vi "PC.vi"() -> ()   [LabVIEW 2016]
uses:
  <vilib>/addons/database/Connection.llb/DB Tools Open Connec (Path).vi
  <vilib>/addons/database/NI_Database_API.lvlib
panel:
  in  "stop 2":bool
  in  "connection information":path
  out "Array 2":dbl[][](array[numeric])
  in  "stop":bool
  in  "kl2":bool
  in  "Reset timer 2":bool
  out "Timer2":u32
  in  "kl1":bool
  in  "Reset timer 1":bool
  out "Timer1":u32
  in  "kl0":bool
  out "Timer0":u32
  in  "Reset timer":bool
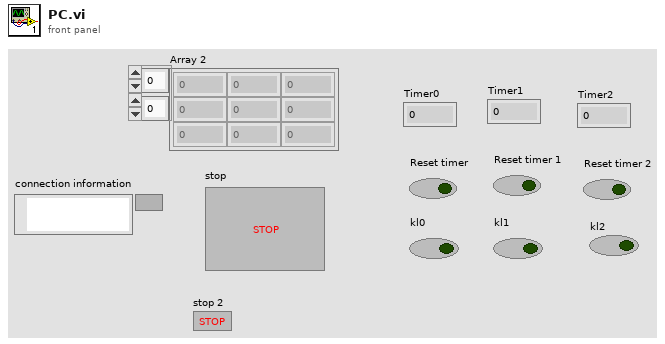
[diagram p1: front panel]
types:
  T1 = cluster{"Place1":string, "Place2":string, "Place3":string}
  T2 = typedef "NI_Database_API.lvlib/Conn ObjectReference.ctl" = refnum<k1>
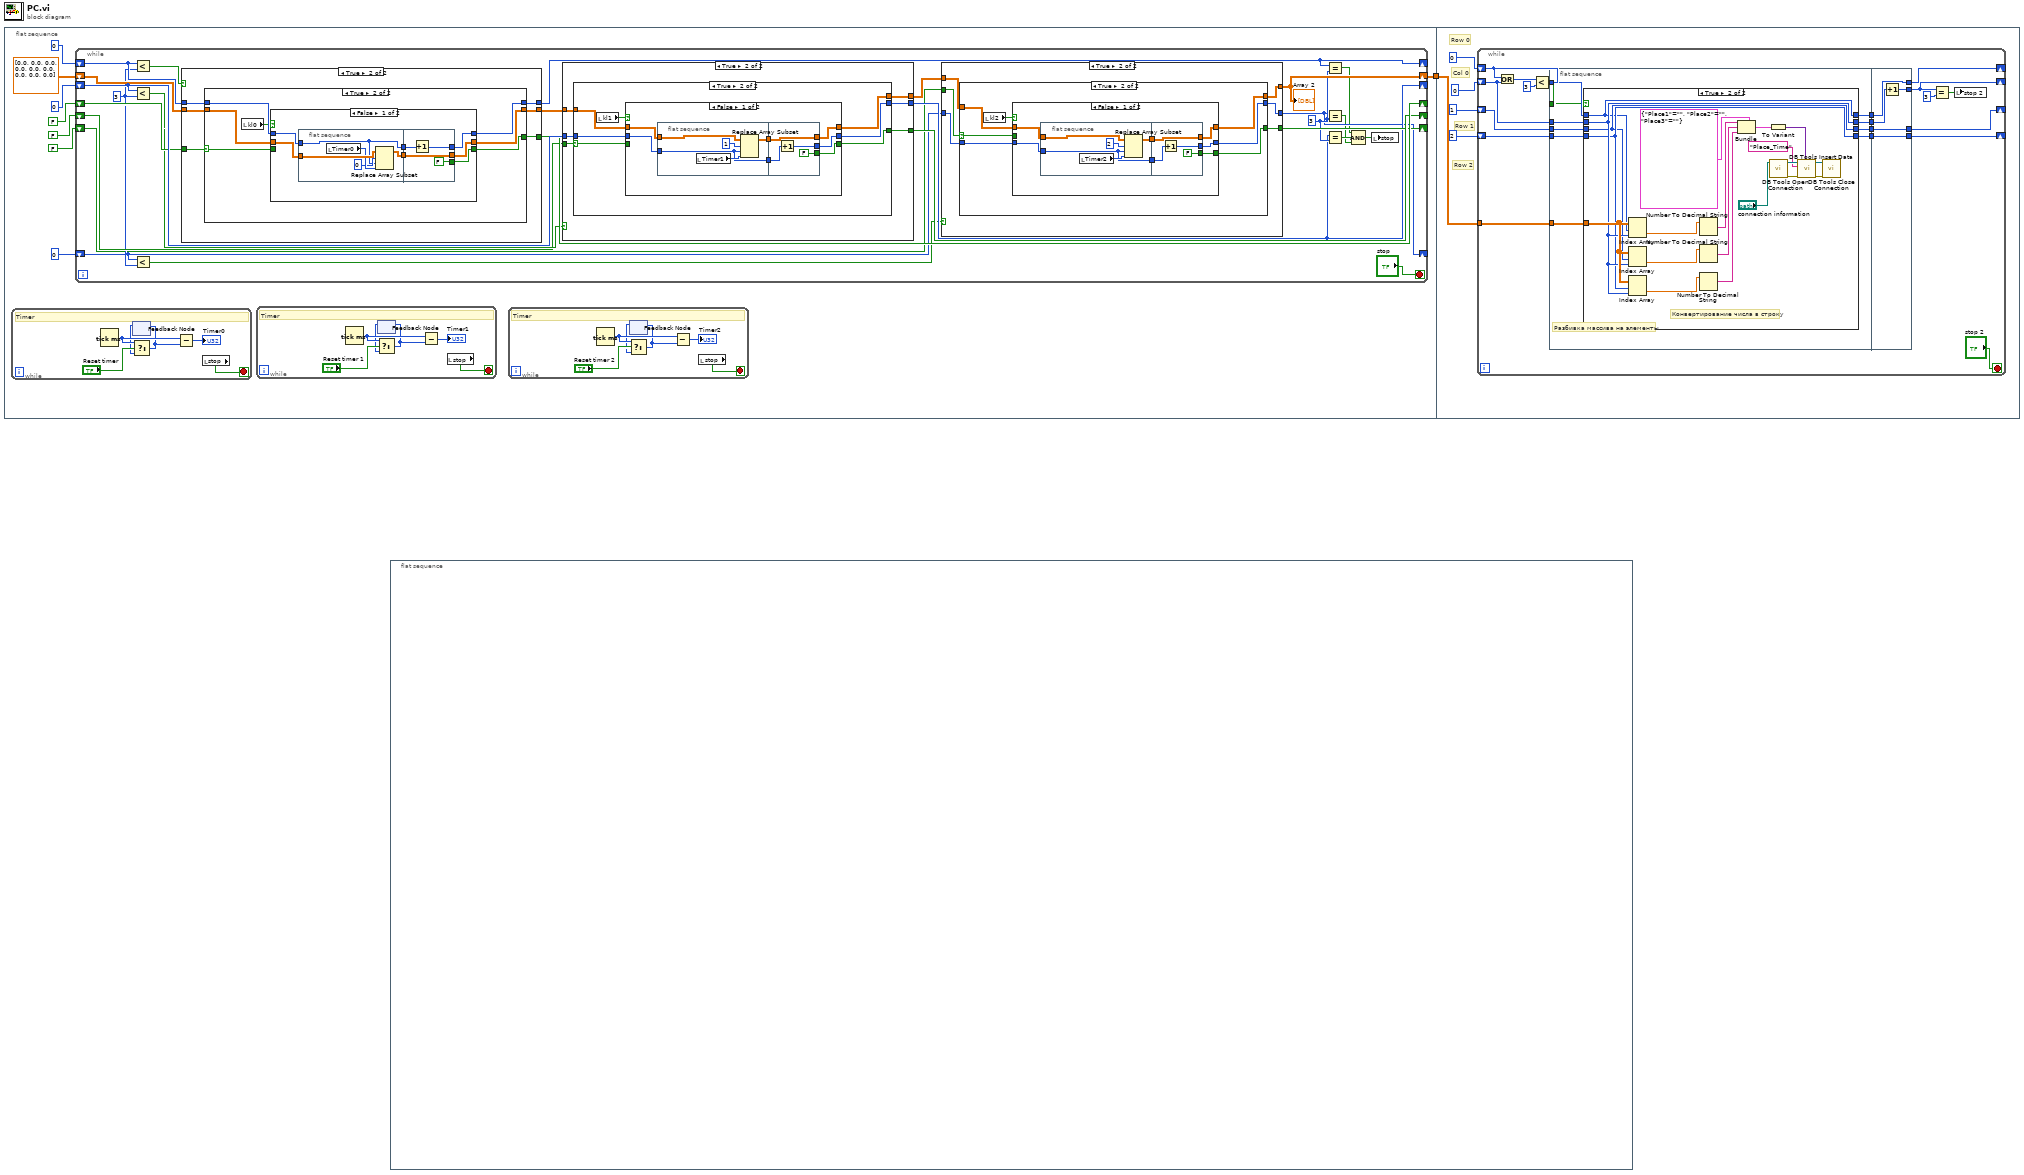
[diagram p0: block diagram]
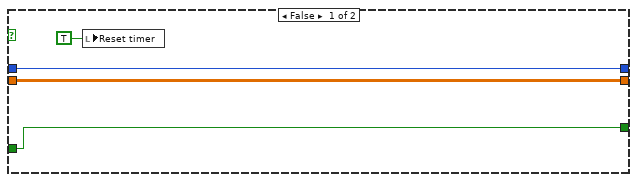
[diagram p2: hidden frame]
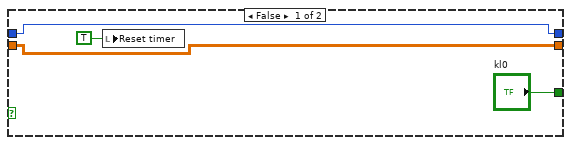
[diagram p3: hidden frame]
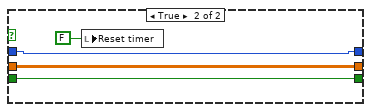
[diagram p4: hidden frame]
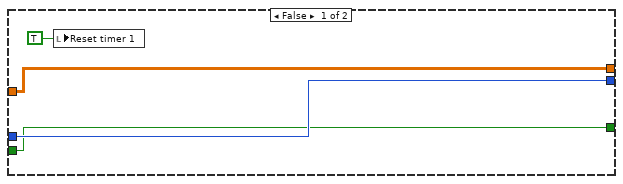
[diagram p5: hidden frame]
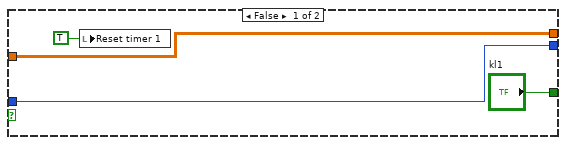
[diagram p6: hidden frame]
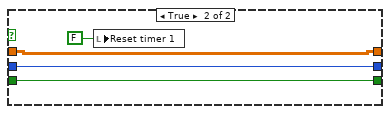
[diagram p7: hidden frame]
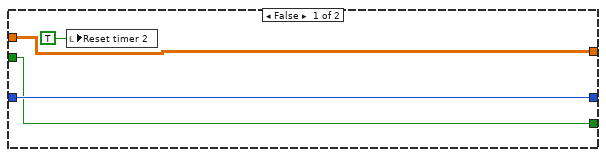
[diagram p8: hidden frame]
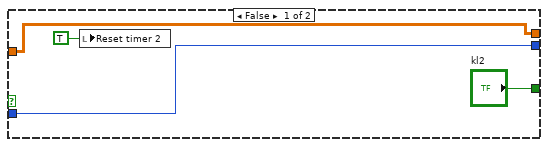
[diagram p9: hidden frame]
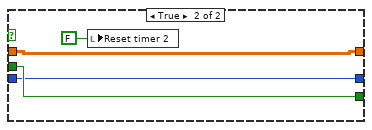
[diagram p10: hidden frame]
diagram:
  n1 = flat-sequence {
    tunnel: [w2] -> w1
    tunnel: w1 -> [w181]
    frame #0 {
      n2 = while {
        stop <- w165 stop-if-true
        # "Timer"
        n3 = Tick Count (ms)() -> (millisecond timer value=w169:u32)
        n4 = feedback #1() -> (w166:u32)  [unwired: 1 in]
        n5 = Select(t=w169, s="Reset timer", f=w166) -> (s? t:f=w167:u32)
        n6 = feedback-in #1(w167) -> ()
        n7 = Subtract(x=w169, y=w167) -> (x-y=→"Timer0":u32)
        n8 = local read "stop"() -> (w165:bool)
      }
      n9 = while {
        shift-right: [w37] -> _
        shift-left: FALSE -> [w25]
        shift-right: [w31] -> _
        shift-left: 0 -> [w41]
        shift-right: [w34] -> w2
        shift-left: dbl[][] [[0.0, 0.0, 0.0], [0.0, 0.0, 0.0], [0.0, 0.0, 0.0]] ("Array") -> [w40]
        shift-right: [w30] -> _
        shift-left: 0 -> [w39]
        shift-right: [w36] -> _
        shift-left: FALSE -> [w23]
        shift-right: [w33] -> _
        shift-left: FALSE -> [w20]
        shift-right: [w29] -> _
        shift-left: 0 -> [w21]
        stop <- "stop" stop-if-true
        w32 = 3
        w22 = 3
        n10 = Less?(x=w41, y=w22) -> (x < y?=w26:bool)
        n11 = Less?(x=w39, y=w22) -> (x < y?=w24:bool)
        n12 = Less?(x=w21, y=w22) -> (x < y?=w19:bool)
        n13 = case shown="True" w26 {
          tunnel: w41 -> [w43 w51]
          tunnel: w40 -> [w44 w50]
          tunnel: [w43 w49] -> w31
          tunnel: [w42 w48] -> w37
          tunnel: [w44 w47] -> w38
          tunnel: w25 -> [w42 w46]
          frame False {
            n14 = local write "Reset timer"(TRUE) -> ()
          }
          frame True {
            n15 = case shown="True" w46 {
              selector: w46 -> [_ w61]
              tunnel: w51 -> [w54 w62]
              tunnel: w50 -> [w53 w60]
              tunnel: [w54 w59] -> w49
              tunnel: ["kl0" w58] -> w48
              tunnel: [w53 w57] -> w47
              frame False {
                n16 = local write "Reset timer"(TRUE) -> ()
              }
              frame True {
                n17 = local read "kl0"() -> (w56:bool)
                n18 = case shown="False" w56 {
                  tunnel: w62 -> [w68 w79]
                  tunnel: w61 -> [_ w81]
                  tunnel: w60 -> [w69 w80]
                  tunnel: [w66 w79] -> w59
                  tunnel: [w65 w81] -> w58
                  tunnel: [w63 w80] -> w57
                  frame False {
                    n19 = flat-sequence {
                      tunnel: w69 -> [w74]
                      tunnel: w68 -> [w71]
                      tunnel: [w71] -> w67
                      tunnel: [w70] -> w64
                      tunnel: w67 -> [w78]
                      tunnel: [w77] -> w66
                      tunnel: [FALSE] -> w65
                      tunnel: w64 -> [w75]
                      tunnel: [w75] -> w63
                      frame #0 {
                        n20 = local read "Timer0"() -> (w73:u32)
                        n21 = Replace Array Subset(array=w74, new element=w73, index (row)=0, index (col)=w71) -> (w70:dbl[][])
                      }
                      frame #1 {
                        n22 = Increment(x=w78) -> (x+1=w77:i32)
                      }
                    }
                  }
                  frame True {
                    n23 = local write "Reset timer"(FALSE) -> ()
                  }
                }
              }
            }
          }
        }
        n24 = case shown="True" w24 {
          tunnel: w39 -> [w85 w92]
          tunnel: w38 -> [w84 w91]
          tunnel: [w85 w90] -> w30
          tunnel: [w83 w89] -> w36
          tunnel: [w84 w88] -> w35
          tunnel: w23 -> [w83 w87]
          frame False {
            n25 = local write "Reset timer 1"(TRUE) -> ()
          }
          frame True {
            n26 = case shown="True" w87 {
              selector: w87 -> [_ w99]
              tunnel: w92 -> [w96 w103]
              tunnel: w91 -> [w93 w102]
              tunnel: [w96 w101] -> w90
              tunnel: ["kl1" w97] -> w89
              tunnel: [w93 w100] -> w88
              frame False {
                n27 = local write "Reset timer 1"(TRUE) -> ()
              }
              frame True {
                n28 = local read "kl1"() -> (w98:bool)
                n29 = case shown="False" w98 {
                  tunnel: w103 -> [w109 w123]
                  tunnel: w102 -> [w110 w122]
                  tunnel: [w107 w123] -> w101
                  tunnel: [w105 w122] -> w100
                  tunnel: w99 -> [_ w121]
                  tunnel: [w104 w121] -> w97
                  frame False {
                    n30 = flat-sequence {
                      tunnel: w110 -> [w115]
                      tunnel: w109 -> [w112]
                      tunnel: [w112] -> w108
                      tunnel: [w111] -> w106
                      tunnel: w108 -> [w119]
                      tunnel: [w118] -> w107
                      tunnel: [w117] -> w105
                      tunnel: w106 -> [w117]
                      tunnel: [FALSE] -> w104
                      frame #0 {
                        n31 = local read "Timer1"() -> (w114:u32)
                        n32 = Replace Array Subset(array=w115, new element=w114, index (row)=1, index (col)=w112) -> (w111:dbl[][])
                      }
                      frame #1 {
                        n33 = Increment(x=w119) -> (x+1=w118:i32)
                      }
                    }
                  }
                  frame True {
                    n34 = local write "Reset timer 1"(FALSE) -> ()
                  }
                }
              }
            }
          }
        }
        n35 = case shown="True" w19 {
          tunnel: w35 -> [w125 w133]
          tunnel: [w125 w132] -> w34
          tunnel: w21 -> [w126 w131]
          tunnel: [w124 w130] -> w33
          tunnel: [w126 w129] -> w29
          tunnel: w20 -> [w124 w128]
          frame False {
            n36 = local write "Reset timer 2"(TRUE) -> ()
          }
          frame True {
            n37 = case shown="True" w128 {
              selector: w128 -> [_ w144]
              tunnel: w133 -> [w135 w143]
              tunnel: [w135 w142] -> w132
              tunnel: w131 -> [w134 w141]
              tunnel: ["kl2" w140] -> w130
              tunnel: [w134 w139] -> w129
              frame False {
                n38 = local write "Reset timer 2"(TRUE) -> ()
              }
              frame True {
                n39 = local read "kl2"() -> (w138:bool)
                n40 = case shown="False" w138 {
                  tunnel: w144 -> [_ w164]
                  tunnel: w143 -> [w151 w163]
                  tunnel: [w149 w163] -> w142
                  tunnel: w141 -> [w148 w162]
                  tunnel: [w147 w164] -> w140
                  tunnel: [w145 w162] -> w139
                  frame False {
                    n41 = flat-sequence {
                      tunnel: w151 -> [w156]
                      tunnel: [w155] -> w150
                      tunnel: w148 -> [w152]
                      tunnel: [w152] -> w146
                      tunnel: [w160] -> w149
                      tunnel: w150 -> [w160]
                      tunnel: [FALSE] -> w147
                      tunnel: w146 -> [w158]
                      tunnel: [w157] -> w145
                      frame #0 {
                        n42 = local read "Timer2"() -> (w153:u32)
                        n43 = Replace Array Subset(array=w156, new element=w153, index (row)=2, index (col)=w152) -> (w155:dbl[][])
                      }
                      frame #1 {
                        n44 = Increment(x=w158) -> (x+1=w157:i32)
                      }
                    }
                  }
                  frame True {
                    n45 = local write "Reset timer 2"(FALSE) -> ()
                  }
                }
              }
            }
          }
        }
        "Array 2" <- w34
        n46 = Equal?(x=w31, y=w32) -> (x = y?=w18:bool)
        n47 = Equal?(x=w29, y=w32) -> (x = y?=w16:bool)
        n48 = Equal?(x=w30, y=w32) -> (x = y?=w17:bool)
        n49 = Compound Arithmetic op=AND(w18, w17, w16) -> (w27:bool)
        n50 = local write "stop"(w27) -> ()
      }
      n51 = while {
        stop <- w10 stop-if-true
        # "Timer"
        n52 = Tick Count (ms)() -> (millisecond timer value=w14:u32)
        n53 = feedback #2() -> (w11:u32)  [unwired: 1 in]
        n54 = Select(t=w14, s="Reset timer 1", f=w11) -> (s? t:f=w12:u32)
        n55 = feedback-in #2(w12) -> ()
        n56 = Subtract(x=w14, y=w12) -> (x-y=→"Timer1":u32)
        n57 = local read "stop"() -> (w10:bool)
      }
      n58 = while {
        stop <- w171 stop-if-true
        # "Timer"
        n59 = Tick Count (ms)() -> (millisecond timer value=w175:u32)
        n60 = feedback #3() -> (w172:u32)  [unwired: 1 in]
        n61 = Select(t=w175, s="Reset timer 2", f=w172) -> (s? t:f=w173:u32)
        n62 = feedback-in #3(w173) -> ()
        n63 = Subtract(x=w175, y=w173) -> (x-y=→"Timer2":u32)
        n64 = local read "stop"() -> (w171:bool)
      }
    }
    frame #1 {
      # "Row 2"
      # "Row 1"
      # "Col 0"
      # "Row 0"
      n65 = while {
        tunnel: w181 -> [w200]
        shift-right: [w182] -> _
        shift-left: 0 -> [w199]
        shift-right: [w190] -> _
        shift-left: 0 -> [w198]
        shift-right: [w184] -> _
        shift-left: 1 -> [w186]
        shift-right: [w188] -> _
        shift-left: 2 -> [w187]
        stop <- "stop 2" stop-if-true
        n66 = Or(x=w199, y=w198) -> (x .or. y?=w197:i32)
        n67 = Less?(x=w197, y=3) -> (x < y?=w195:bool)
        n68 = flat-sequence {
          tunnel: w200 -> [w210]
          tunnel: w199 -> [w209]
          tunnel: w198 -> [w208]
          tunnel: w186 -> [w207]
          tunnel: w187 -> [w206]
          tunnel: w195 -> [w205]
          tunnel: [w204] -> w194
          tunnel: [w203] -> w189
          tunnel: [w202] -> w185
          tunnel: [w201] -> w183
          tunnel: w194 -> [w239]
          tunnel: [w238] -> w190
          tunnel: [w237] -> w188
          tunnel: w189 -> [w237]
          tunnel: [w236] -> w184
          tunnel: w185 -> [w236]
          tunnel: [w235] -> w182
          tunnel: w183 -> [w235]
          frame #0 {
            # "Разбивка массива на элементы"
            n69 = case shown="True" w205 {
              tunnel: w210 -> [_ w234]
              tunnel: w209 -> [w214 w215]
              tunnel: w208 -> [w213 w218]
              tunnel: w207 -> [w212 w216]
              tunnel: w206 -> [w211 w217]
              tunnel: [w213 w218] -> w204
              tunnel: [w211 w217] -> w203
              tunnel: [w212 w216] -> w202
              tunnel: [w214 w215] -> w201
              frame False {
              }
              frame True {
                # "Конвертирование числа в строку"
                n70 = Index Array(array=w234, index (row)=w215, index (col)=w218) -> (element=w231:dbl)
                n71 = Index Array(array=w234, index (row)=w216, index (col)=w218) -> (element=w232:dbl)
                n72 = Index Array(array=w234, index (row)=w217, index (col)=w218) -> (element=w233:dbl)
                n73 = Number To Decimal String(number=w231) -> (decimal integer string=w229:string)  [unwired: 1 in]
                n74 = Number To Decimal String(number=w232) -> (decimal integer string=w228:string)  [unwired: 1 in]
                n75 = Number To Decimal String(number=w233) -> (decimal integer string=w227:string)  [unwired: 1 in]
                n76 = Bundle(cluster=T1 {"Place1"="", "Place2"="", "Place3"=""}, "Place1"=w229, "Place2"=w228, "Place3"=w227) -> (w226:T1)
                n77 = To Variant(anything=w226) -> (Variant=w219:variant)
                n78 = call-poly <vilib>:"DB Tools Open Connection.vi"("connection information"="connection information") -> ("error out"=w222:errorcluster, "connection reference"=w223:T2)  [unwired: 7 in]
                n79 = call <vilib>:"DB Tools Insert Data.vi"("data"=w219, "error in (no error)"=w222, "table"="Place_Time", "connection reference"=w223) -> ("error out"=w225:errorcluster, "connection reference out"=w224:T2)  [unwired: 6 in]
                n80 = call <vilib>:"DB Tools Close Connection.vi"("error in (no error)"=w225, "connection reference"=w224) -> ()  [unwired: 5 in, 1 out]
              }
            }
          }
          frame #1 {
            n81 = Increment(x=w239) -> (x+1=w238:i32)
          }
        }
        n82 = Equal?(x=w190, y=3) -> (x = y?=w191:bool)
        n83 = local write "stop 2"(w191) -> ()
      }
    }
  }
  n84 = flat-sequence {
    frame #0 {
    }
  }
